vi "3.1.1-VectorNav Parse Reply.vi"(11 "Input String":string="$VNRRG,08,+000.00,+000.00,+000.00*00") -> (1 "Data":dbl[](array[numeric]), 2 "Register":T1, 3 "Header":string)   [LabVIEW 2010]
uses:
  3.1.1-VectorNav Registers.ctl
  <vilib>/regexp/Match Regular Expression.xnode
  3.1.1-VectorNav Data.ctl
  3.0-Global.vi
panel:
  out "Async Data Output Freq":dbl
  out "Async Data Output Type":dbl
  out "Serial Baud Rate":dbl
  out "Firmware Version":dbl
  out "Serial Number":dbl
  out "Hardware Revision":dbl
  out "Model":string
  out "Roll":dbl
  out "Pitch":dbl
  out "Yaw":dbl
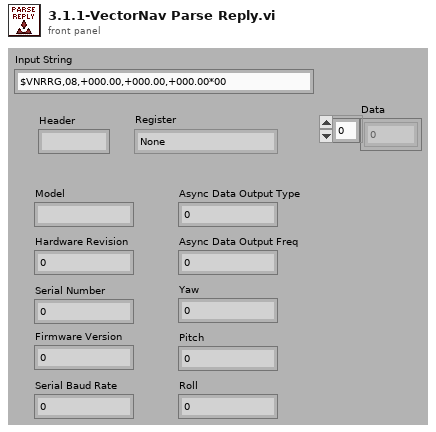
[diagram p1: front panel]
types:
  T1 = typedef "3.1.1-VectorNav Registers.ctl" = enum16{"None", "Model Number", "Hardware Revision", "Serial Number", "Firmware Version", "Serial Baud Rate", "Async Data Output Type", "Async Data Output Freq", "Attitude (Yaw, Pitch, Roll)", "Attitude (Quaternion)"}
  T2 = typedef "3.1.1-VectorNav Data.ctl" = cluster{"Yaw":dbl, "Pitch":dbl, "Roll":dbl}
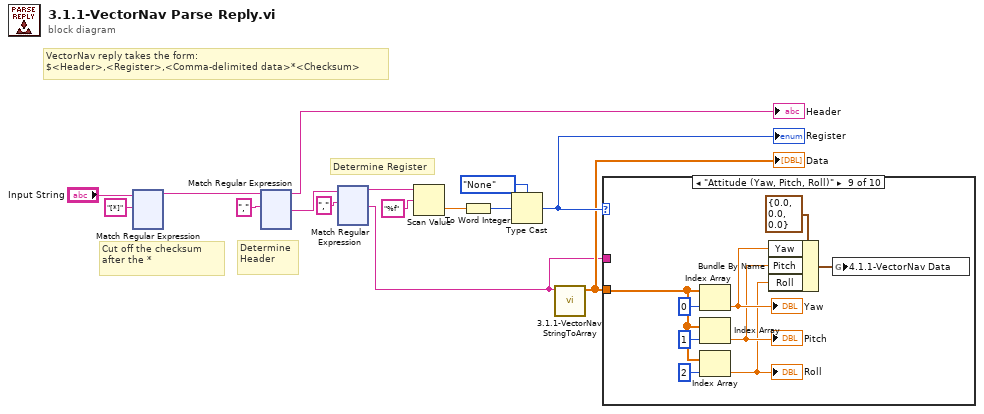
[diagram p0: block diagram]
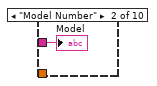
[diagram p3: hidden frame]
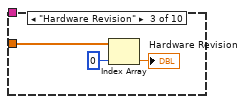
[diagram p4: hidden frame]
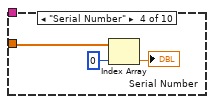
[diagram p5: hidden frame]
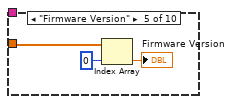
[diagram p6: hidden frame]
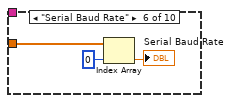
[diagram p7: hidden frame]
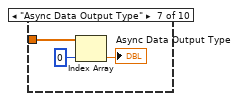
[diagram p8: hidden frame]
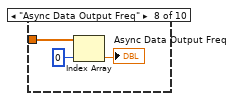
[diagram p9: hidden frame]
diagram:
  # "VectorNav reply takes the form:\n$<Header>,<Register>,<Comma-delimited data>*<Checksum>"
  # "Determine Header"
  # "Determine Register"
  # "Cut off the checksum after the *"
  n1 = xnode "Match Regular Expression"("input string"="Input String", "regular expression"="[*]") -> ("before match"=w8:string)  [unwired: 4 in, 4 out]
  n2 = xnode "Match Regular Expression"("input string"=w8, "regular expression"=",") -> ("before match"=→"Header":string, "after match"=w10:string)  [unwired: 4 in, 3 out]
  n3 = xnode "Match Regular Expression"("input string"=w10, "regular expression"=",") -> ("before match"=w1:string, "after match"=w2:string)  [unwired: 4 in, 3 out]
  n4 = Scan Value(string=w1, format string="%f") -> (value=w5:dbl)  [unwired: 1 in, 1 out]
  n5 = To Word Integer(number=w5) -> (16bit integer=w6:i16)
  n6 = Type Cast(type=3.1.1-VectorNav_Registers."None" ("VectorNav Registers"), x=w6) -> (*(type *) &x=w4:T1)
  "Register" <- w4
  n7 = call "3.1.1-VectorNav StringToArray.vi"("String"=w2) -> ("Array"=w3:dbl[])  [unwired: 10 in]
  "Data" <- w3
  n8 = case shown="\"Attitude (Yaw, Pitch, Roll)\"" w4 {
    tunnel: w2 -> [_ w16 _ _ _ _ _ _ _ _]
    tunnel: w3 -> [_ _ w17 w20 w23 w26 w29 w32 w40 _]
    frame "None", Default {
    }
    frame "Model Number" {
      "Model" <- w16
    }
    frame "Hardware Revision" {
      n9 = Index Array(array=w17, index=0) -> (element=→"Hardware Revision":dbl)
    }
    frame "Serial Number" {
      n10 = Index Array(array=w20, index=0) -> (element=→"Serial Number":dbl)
    }
    frame "Firmware Version" {
      n11 = Index Array(array=w23, index=0) -> (element=→"Firmware Version":dbl)
    }
    frame "Serial Baud Rate" {
      n12 = Index Array(array=w26, index=0) -> (element=→"Serial Baud Rate":dbl)
    }
    frame "Async Data Output Type" {
      n13 = Index Array(array=w29, index=0) -> (element=→"Async Data Output Type":dbl)
    }
    frame "Async Data Output Freq" {
      n14 = Index Array(array=w32, index=0) -> (element=→"Async Data Output Freq":dbl)
    }
    frame "Attitude (Yaw, Pitch, Roll)" {
      n15 = Index Array(array=w40, index=0) -> (element=w37:dbl)
      "Yaw" <- w37
      n16 = Index Array(array=w40, index=1) -> (element=w36:dbl)
      "Pitch" <- w36
      n17 = Index Array(array=w40, index=2) -> (element=w35:dbl)
      "Roll" <- w35
      n18 = Bundle By Name(cluster=T2 {"Yaw"=0.0, "Pitch"=0.0, "Roll"=0.0} ("VectorNav Data"), "Yaw"=w37, "Pitch"=w36, "Roll"=w35) -> (w39:T2)
      n19 = global write "3.0-Global.vi" "4.1.1-VectorNav Data"(w39) -> ()
    }
    frame "Attitude (Quaternion)" {
    }
  }
